vi "Read File Refnum.vi"(11 "Text File Sink in":refnum<class "Text File Sink.lvclass">) -> (2 "File Refnum":refnum<file>, 3 "Text File Sink out":refnum<class "Text File Sink.lvclass">)   [LabVIEW 2016, in "Stream Log.lvlib" / "Text File Sink.lvclass"]
uses:
  <userlib>/Composed Systems/Stream/Log/Text File Sink/Text File Sink.lvclass
  <userlib>/Composed Systems/Stream/Log/Text File Sink/Text File Sink.lvclass/Text File Sink.ctl
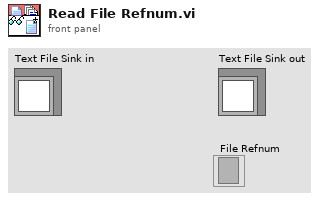
[diagram p1: front panel]
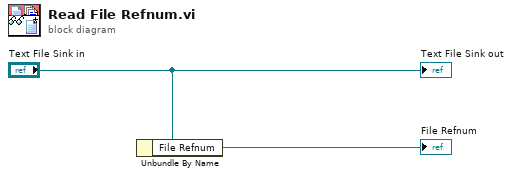
[diagram p0: block diagram]
diagram:
  n1 = Unbundle By Name("Text File Sink in") -> ("File Refnum"=→"File Refnum":refnum<file>)
  "Text File Sink out" <- "Text File Sink in"
